vi "Globals.vi"() -> ()   [LabVIEW 2020]
panel:
  in  "main vi reference":refnum<vi>
  in  "current data":dbl[][](array[numeric])
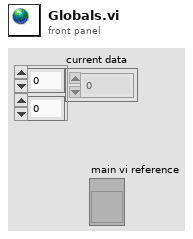
[diagram p1: front panel]
diagram:
